vi "BB_Label_Horiz.vi"(7 "Limit Passed":bool, 8 "Limits":dbl[](array[numeric]), 9 "Scores":dbl[](array[numeric]), 10 "Bounding Box":T1, 11 "image in":T2) -> (0 "Limits Out":dbl[](array[numeric]), 1 "Scores Out":dbl[](array[numeric]), 2 "Bounding BoxOut":T1, 3 "image out":T2)   [LabVIEW 2015]
doc: "Add a rectangle border around the inside and outside of what is believed to be the reflective tape. Also place the color coded scores next to all of the large blobs being processed."
uses:
  <vilib>/vision/Image Controls.llb/IMAQ Image.ctl
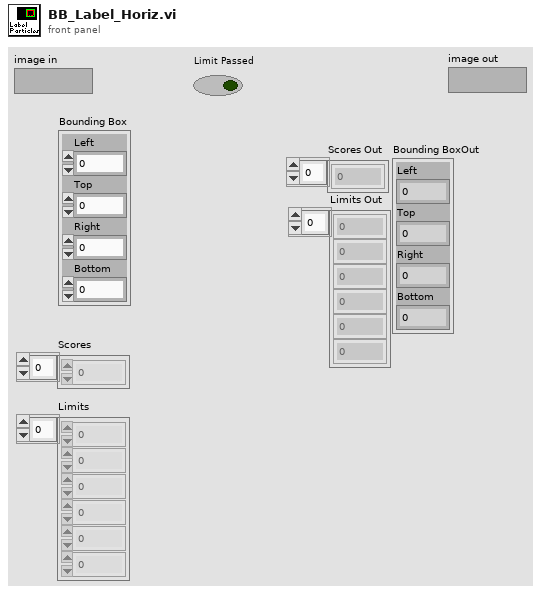
[diagram p1: front panel]
types:
  T1 = cluster{"Left":dbl, "Top":dbl, "Right":dbl, "Bottom":dbl}
  T2 = typedef "IMAQ Image.ctl" = refnum<image>
  T3 = cluster{"Desired Font (Application)":enum16{"User-specified Font", "Application Font", "System Font", "Dialog Font"}, "[User-specified Font]":cluster{"Font Name":string, "Size":i16, "Strikeout?":bool, "Italic?":bool, "Underline?":bool, "Outline?":bool, "Shadow?":bool, "Bold?":bool, "Rotation Angle":dbl}, "Horizontal Alignment":i16, "Vertical Alignment":i16}
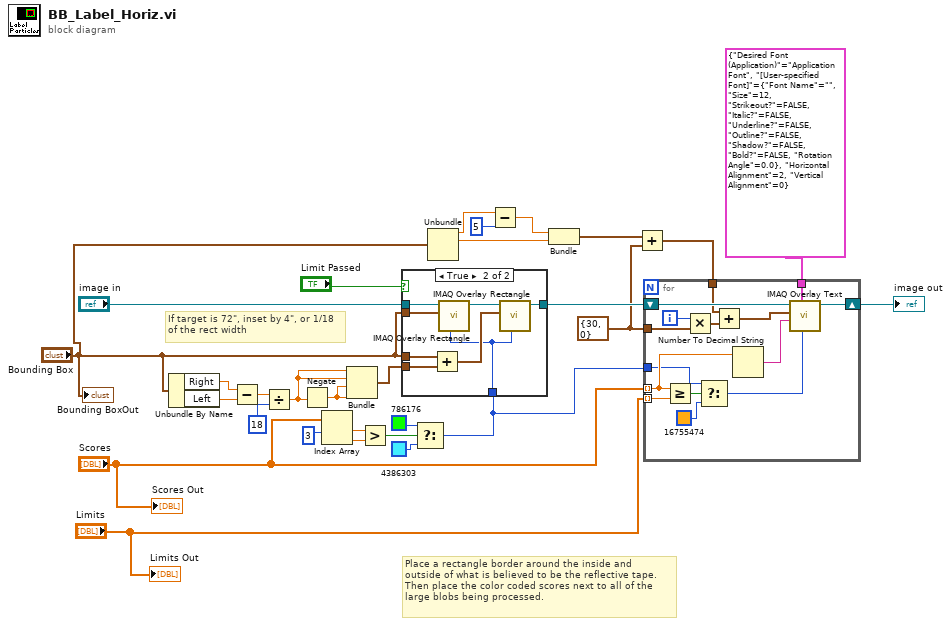
[diagram p0: block diagram]
diagram:
  w18 = cluster{i32, i32} {30, 0}
  # "Place a rectangle border around the inside and\noutside of what is believed to be the reflective tape.\nThen place the color coded scores next to all of the\nlarge blobs being processed."
  # "If target is 72\", inset by 4\", or 1/18\nof the rect width"
  n1 = Unbundle By Name("Bounding Box") -> ("Right"=w16:dbl, "Left"=w15:dbl)
  n2 = Subtract(x=w16, y=w15) -> (x-y=w13:dbl)
  n3 = Divide(x=w13, y=18) -> (x/y=w11:dbl)
  n4 = Negate(x=w11) -> (-x=w17:dbl)
  n5 = Index Array(array="Scores", index #1=3 ("length")) -> (element #1=w6:dbl, element #2=w5:dbl)  [unwired: 1 in]
  n6 = Bundle(w11, w11, w17, w17) -> (w14:cluster{dbl, dbl, dbl, dbl})  [unwired: 1 in]
  n7 = Greater?(x=w6, y=w5) -> (0:w4:bool)
  n8 = Select(t=u32 786176 ("Color"), s=w4, f=u32 4386303 ("Color")) -> (s? t:f=w1:u32)
  n9 = case shown="True" "Limit Passed" {
    tunnel: "image in" -> [w30 w38]
    tunnel: "Bounding Box" -> [_ w37]
    tunnel: "Bounding Box" -> [_ w35]
    tunnel: [w30 w33] -> w25
    tunnel: w14 -> [_ w32]
    tunnel: w1 -> [_ w31]
    frame False {
    }
    frame True {
      n10 = Add(x=w35, y=w32) -> (x+y=w34:cluster{dbl, dbl, dbl, dbl})
      n11 = call "IMAQ Overlay Rectangle"("Color"=w31, "Rectangle"=w37, "Image"=w38) -> ("Image Out"=w36:T2)  [unwired: 3 in, 5 out]
      n12 = call "IMAQ Overlay Rectangle"("Color"=w31, "Rectangle"=w34, "Image"=w36) -> ("Image Out"=w33:T2)  [unwired: 3 in, 5 out]
    }
  }
  n13 = Unbundle("Bounding Box") -> ("Left"=w23:dbl, "Top"=w24:dbl)  [unwired: 2 out]
  n14 = Subtract(x=w23, y=5) -> (x-y=w22:dbl)
  n15 = Bundle(w22, "Top"=w24) -> (w20:cluster{dbl, "Top":dbl})  [unwired: 1 in]
  n16 = Add(x=w20, y=w18) -> (x+y=w19:cluster{dbl, dbl})
  n17 = for {
    shift-right: [w52] -> w28
    shift-left: w25 -> [w53]
    tunnel: "Scores" -> [w46] mode=indexing
    tunnel: "Limits" -> [w51] mode=indexing
    tunnel: w18 -> [w43]
    tunnel: w19 -> [w42]
    tunnel: T3 {"Desired Font (Application)"=enum."Application Font", "[User-specified Font]"={"Font Name"="", "Size"=12, "Strikeout?"=FALSE, "Italic?"=FALSE, "Underline?"=FALSE, "Outline?"=FALSE, "Shadow?"=FALSE, "Bold?"=FALSE, "Rotation Angle"=0.0}, "Horizontal Alignment"=2, "Vertical Alignment"=0} ("Font, Size & Style") -> [w40]
    tunnel: w1 -> [w39]
    i -> [w45]
    n18 = Greater Or Equal?(x=w46, y=w51) -> (x >= y?=w50:bool)
    n19 = Multiply(x=w45, y=w43) -> (x*y=w44:cluster{i32, i32})
    n20 = Select(t=w39, s=w50, f=u32 16755474 ("Color")) -> (s? t:f=w47:u32)
    n21 = Add(x=w42, y=w44) -> (x+y=w41:cluster{dbl, dbl})
    n22 = Number To Decimal String(number=w46) -> (decimal integer string=w48:string)  [unwired: 1 in]
    n23 = call "IMAQ Overlay Text"("Text Color (black)"=w47, "Font, Size & Style"=w40, "String"=w48, "Origin"=w41, "Image"=w53) -> ("Image Out"=w52:T2)  [unwired: 5 in, 1 out]
  }
  "image out" <- w28
  "Scores Out" <- "Scores"
  "Limits Out" <- "Limits"
  "Bounding BoxOut" <- "Bounding Box"
